vi "ritter sample 1.vi"() -> ()   [LabVIEW 2023]
doc: "Each half second this this program reads the current flow and accumulated volume."
uses:
  Type Definitions/Input Parameters.ctl
  Type Definitions/Full Data.ctl
  Type Definitions/EDU 32 FP Data Cluster.ctl
  <vilib>/Platform/TimedLoop/XDataNode/timing_clust.ctl
  <vilib>/Platform/TimedLoop/XDataNode/nitl_modes.ctl
  <vilib>/Platform/TimedLoop/XDataNode/wakeup.ctl
  <vilib>/platform/TimedLoop/XDataNode/XDataNode.xnode
  <vilib>/Platform/TimedLoop/XDataNode/XDNodeRunTimeDep.lvlib
panel:
  in  "Tab Control 2":enum32{"Page 1", "Page 2"}(tab)
  out "Full Data Set":T1 {"EDU 32 FP- Data"."English"."Gas Flow Rate (cuft/hr)-Raw" format="%.2f"; "EDU 32 FP- Data"."Metric"."Gas Flow Rate (L/hr)-Raw" format="%.2f"}
  in  "Input Parameters":T3={"Barometric Pressure (inHG)"=0.0, "Gas Pressure (in WC)"=0.0, "Gas Temperature (°F)"=0.0, "Standard Pressure (in HG)"=30.0, "Meter Type"=enum."Wet Meter"}
  out "Correction Factor":dbl
  out "Pressure Correction Factor":dbl
  out "Temperature Correction Factor":dbl
  out "Totalized Flow (L)-Corrected":dbl format="%.3f"
  out "Gas Flow Rate (L/hr)-Corrected":dbl format="%.3f"
  in  "Tab Control":enum32{"Main Screen"}(tab)
  in  "Test Point (Nominal)":T4(ring)
  out "Elapsed Time (Hour)":dbl format="%.2f"
  out "Totalization (L) Snapshot 1":dbl format="%.3f"
  out "Gas Flow Rate (L/hr) Snapshot 1":dbl format="%.3f"
  in  "Timer Snapshot 1(Minutes)":dbl=15.0 format="%.2f"
  out "Elapsed Time (Minute)":dbl format="%.2f"
  in  "Ritter VISA":refnum<visa-resource-name>="COM10"
  out "Totalized Flow (L)-Display":dbl format="%.3f"
  out "Gas Flow Rate (L/hr)-Display":dbl format="%.1f"
  out "Gas Flow Rate (L/hr)-Uncorrected-Calibration":dbl format="%.3f"
  in  "Reset":bool
  in  "Exit":bool
  # "STP Correction\nStandard Temperature = 60°F\nStandard Pressure = 30 in HG"
  # "Calculated Correction Factors"
  # "Flow Rate Calibration - Uncorrected"
  # "or"
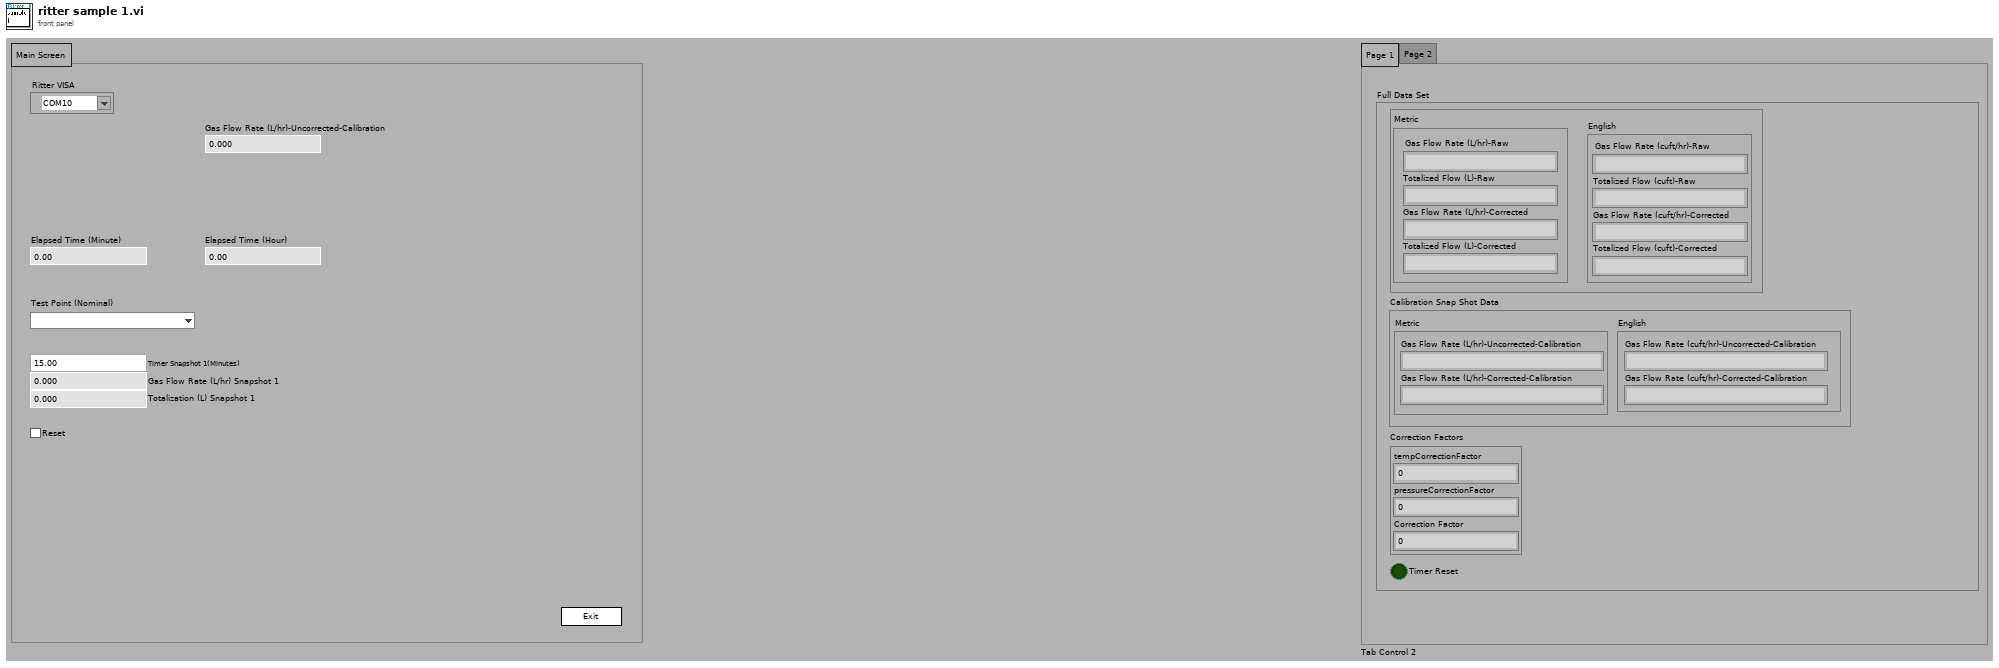
[diagram p1: front panel]
types:
  T1 = typedef "Full Data.ctl" = cluster{"EDU 32 FP- Data":T2, "Calibration Snap Shot Data":cluster{"Metric":cluster{"Gas Flow Rate (L/hr)-Corrected-Calibration":dbl, "Gas Flow Rate (L/hr)-Uncorrected-Calibration":dbl}, "English":cluster{"Gas Flow Rate (cuft/hr)-Corrected-Calibration":dbl, "Gas Flow Rate (cuft/hr)-Uncorrected-Calibration":dbl}}, "Correction Factors":cluster{"tempCorrectionFactor":dbl, "pressureCorrectionFactor":dbl, "Correction Factor":dbl}, "Timer Reset":bool}
  T2 = typedef "EDU 32 FP Data Cluster.ctl" = cluster{"Metric":cluster{"Totalized Flow (L)-Raw":dbl, "Gas Flow Rate (L/hr)-Raw":dbl, "Totalized Flow (L)-Corrected":dbl, "Gas Flow Rate (L/hr)-Corrected":dbl}, "English":cluster{"Totalized Flow (cuft)-Raw":dbl, "Gas Flow Rate (cuft/hr)-Raw":dbl, "Totalized Flow (cuft)-Corrected":dbl, "Gas Flow Rate (cuft/hr)-Corrected":dbl}}
  T3 = typedef "Input Parameters.ctl" = cluster{"Barometric Pressure (inHG)":dbl, "Gas Pressure (in WC)":dbl, "Gas Temperature (°F)":dbl, "Standard Pressure (in HG)":dbl, "Meter Type":enum16{"Wet Meter", "Dry Meter"}}
  T4 = enum16{"", "14 L/hr @ 30 Minutes", "460 L/hr @ 15 Minutes", "900 L/hr @ 15 Minutes", "1100 L/hr @ 15 Minutes", "1100 L/hr @ 100 Minutes", "1300 L/hr @ 15 Minutes"}
  T5 = typedef "XDNodeRunTimeDep.lvlib/timing_clust.ctl" = cluster{"Expected End [f-1]":u64, "Actual End [f-1]":u64, "Finished Late? [f-1]":bool, "Expected End [i-1]":u64, "Actual End [i-1]":u64, "Finished Late? [i-1]":bool, "Expected Start [i]":u64, "Actual Start [i]":u64, "Expected Start [f]":u64, "Actual Start [f]":u64, "Source Name":string, "Structure Name":string, "Period":i64, "Deadline":i64, "Offset":i64, "Start":i64, "Priority":i32, "Timeout":i32, "Mode":T6, "Wakeup Reason":T7, "Error":errorcluster, "Source Type":string, "Secondary Source Type":string, "Global End Time":u64, "Global Start Time":u64, "Frame Duration":u64, "Iteration Duration":u64, "Assigned CPU":i32, "I/O Scan Engine Mode":u32}
  T6 = typedef "XDNodeRunTimeDep.lvlib/nitl_modes.ctl" = enum32{"No Change", "Process missed periods, maintain original phase", "Discard missed periods, maintain original phase", "Process missed periods, ignore original phase", "Discard missed periods, ignore original phase"}
  T7 = typedef "XDNodeRunTimeDep.lvlib/wakeup.ctl" = enum32{"Normal", "Aborted", "Asynchronous wakeup", "Timing source error", "Timed loop error", "Timeout"}
  T8 = enum32{"Invalid", "Standard", "Closed", "Hidden", "Minimized", "Maximized"}
  T9 = enum32{"invalid app kind", "Development System", "Run Time System", "Student Edition", "Embedded LabVIEW", "Evaluation", "Custom"}
  T10 = cluster{"Core":cluster{"Current VI Reference":refnum<vi>, "Close Panel on Exit?":bool}, "Ritter VISA":refnum<visa-resource-name>, "Full Data Set":T1}
  T11 = cluster{"Current VI Reference":refnum<vi>, "Close Panel on Exit?":bool}
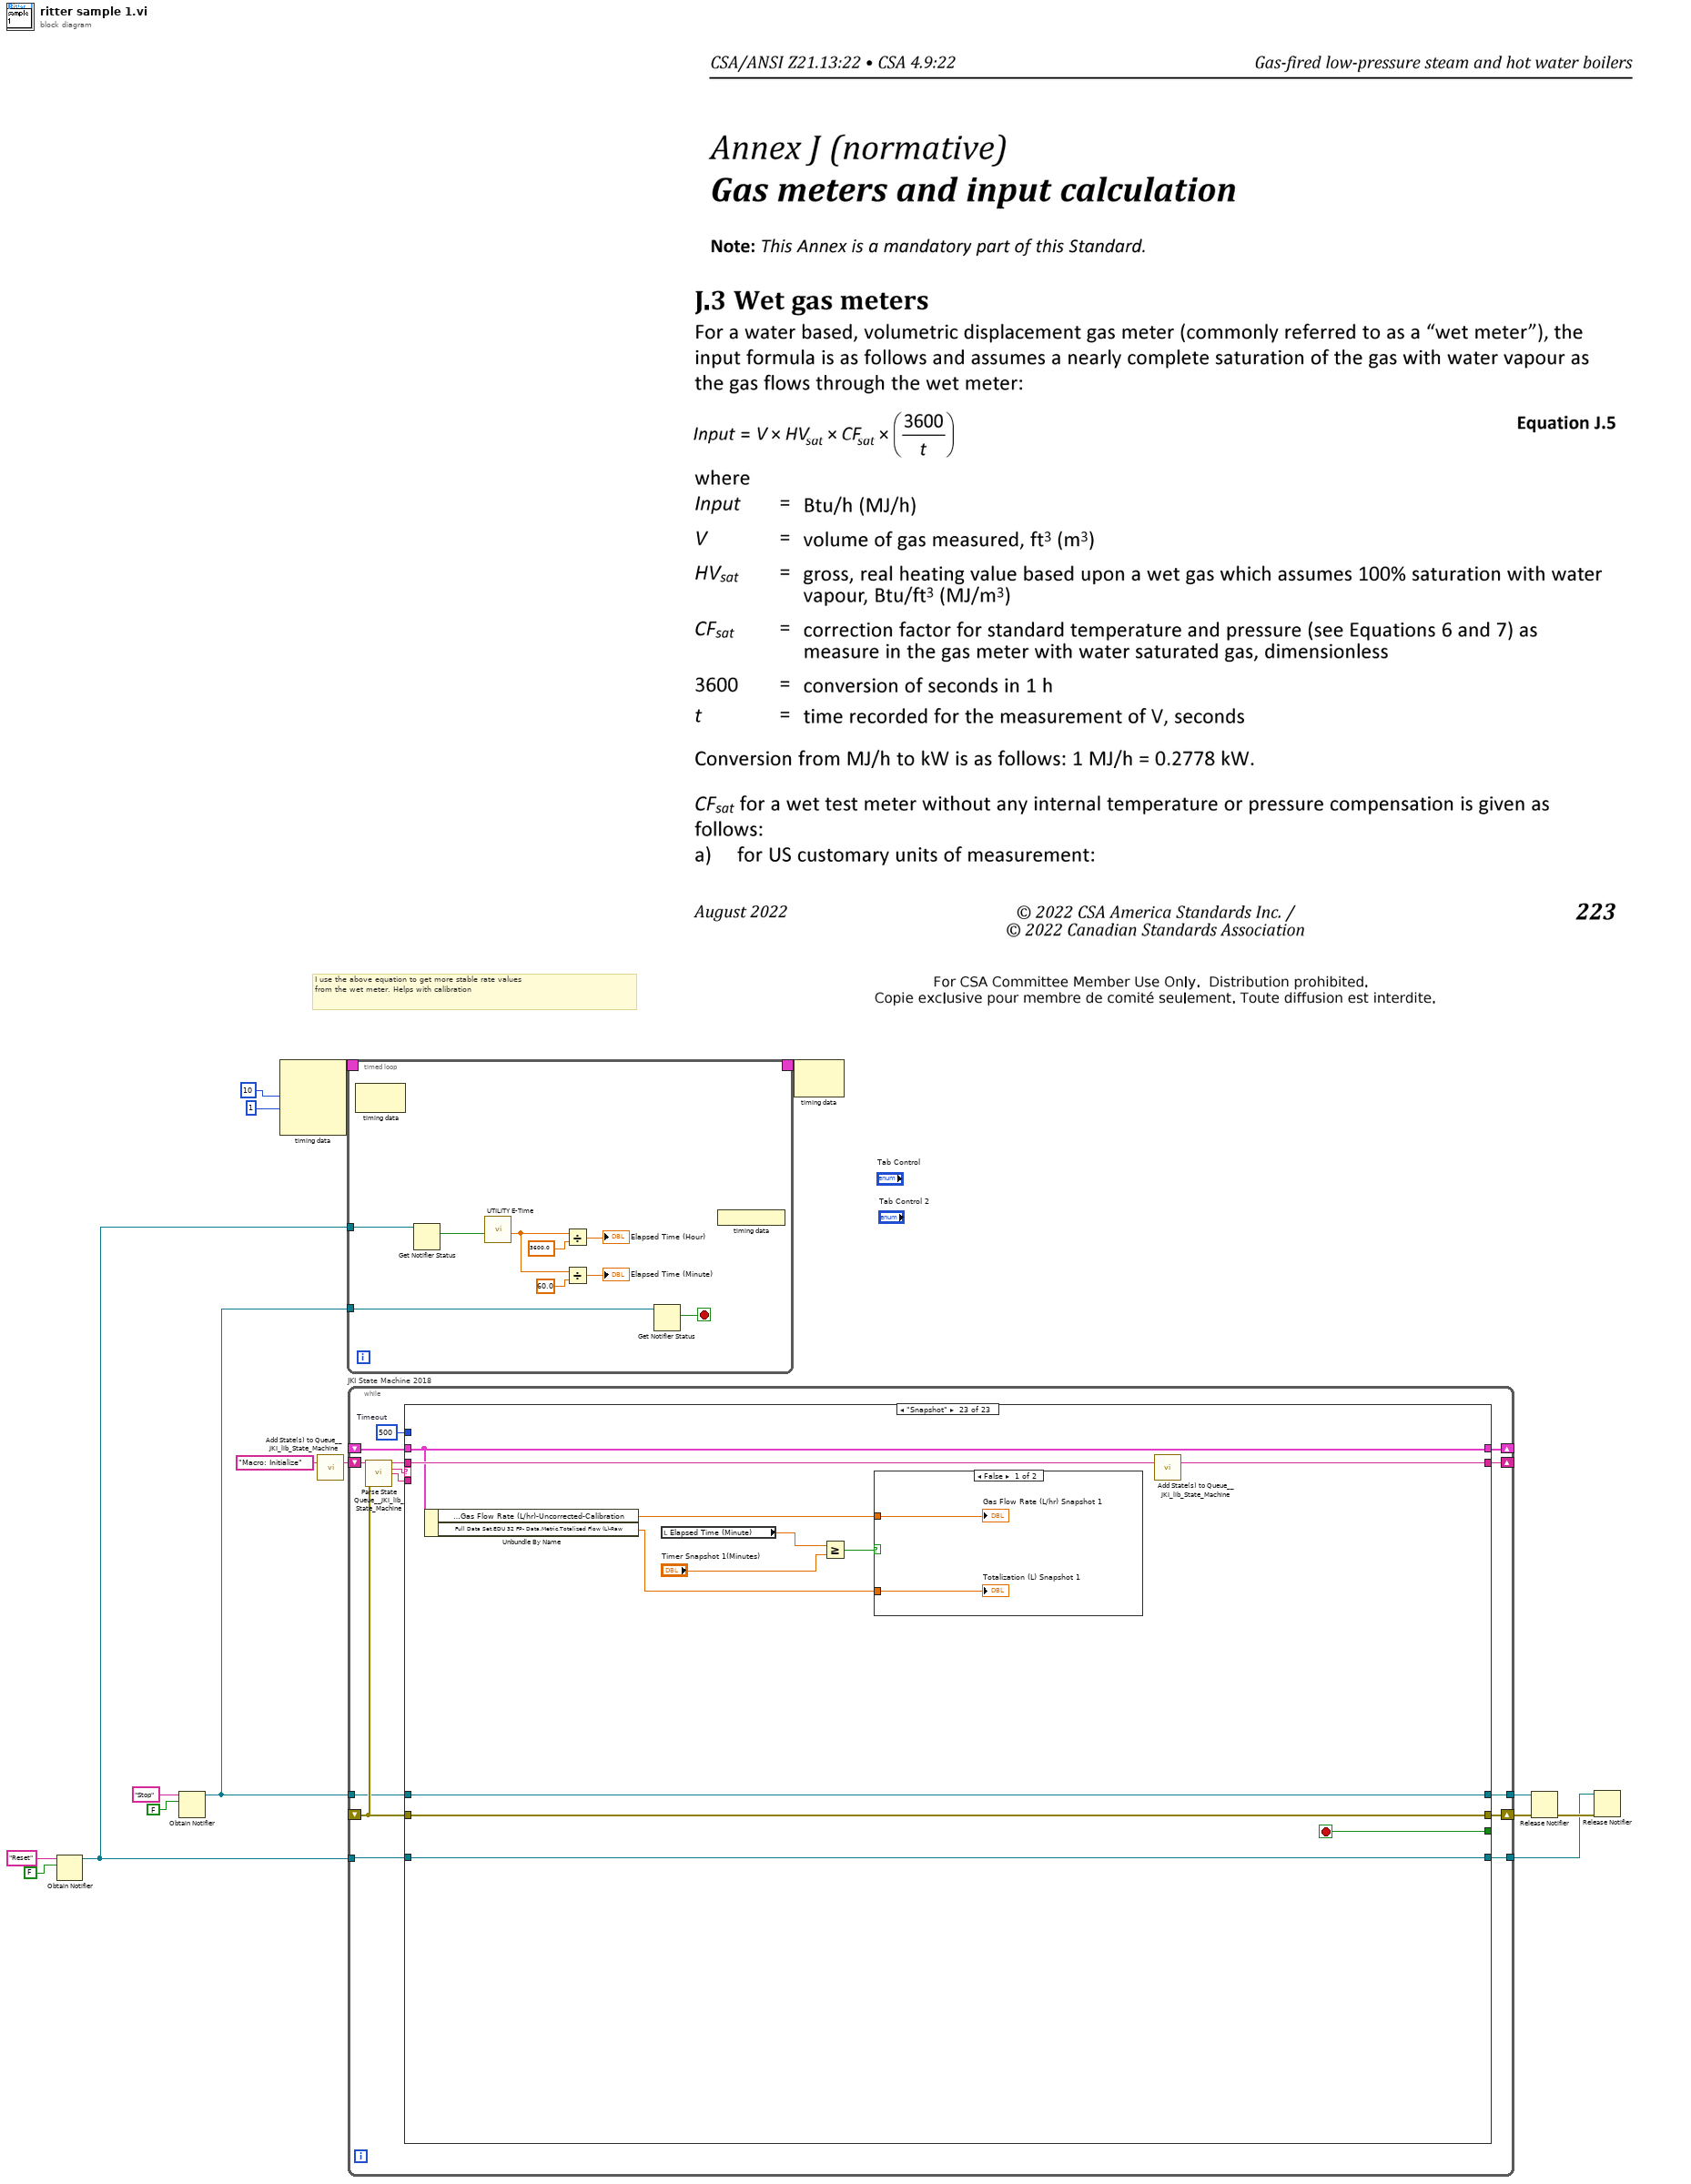
[diagram p0: block diagram]
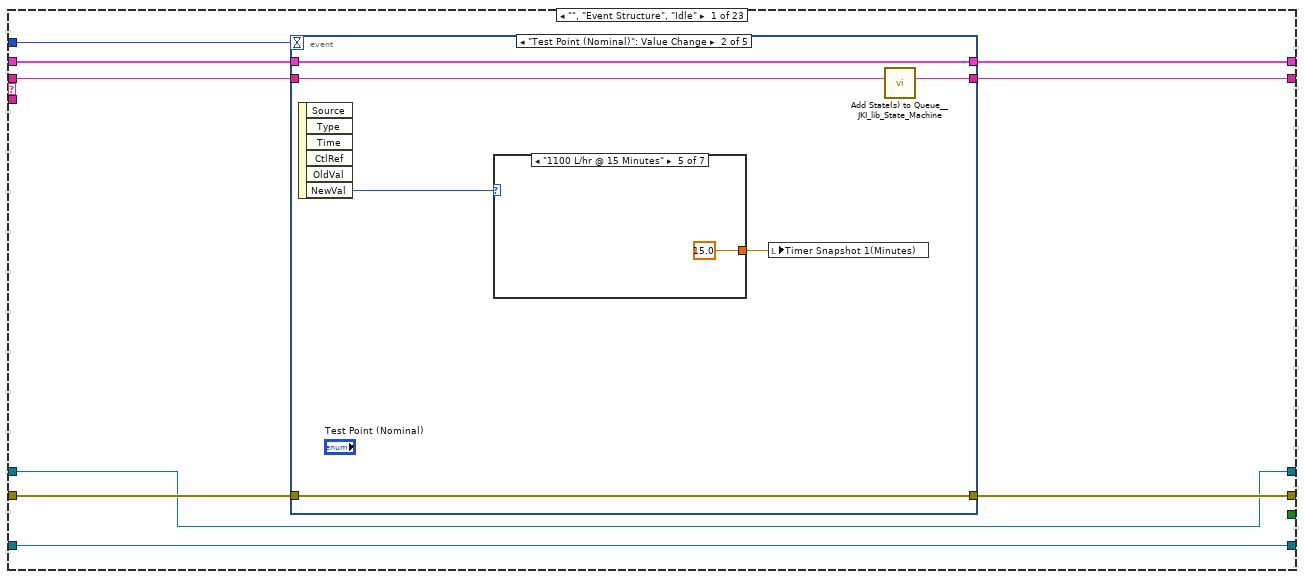
[diagram p2: hidden frame]
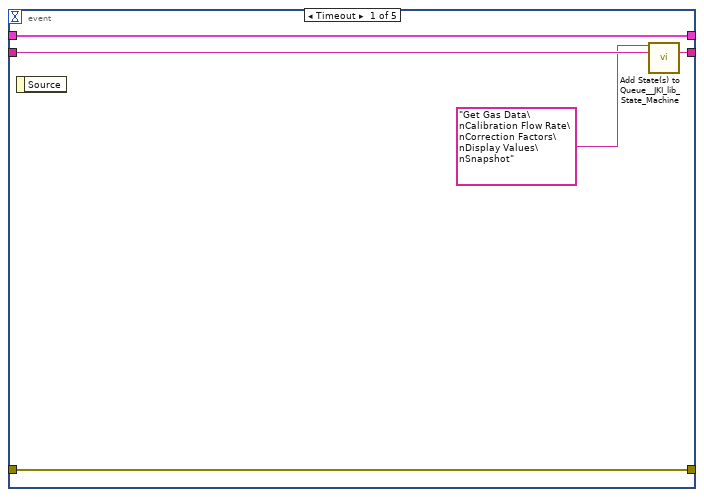
[diagram p3: hidden frame]
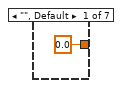
[diagram p4: hidden frame]
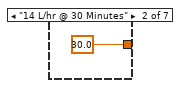
[diagram p5: hidden frame]
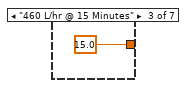
[diagram p6: hidden frame]
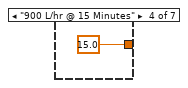
[diagram p7: hidden frame]
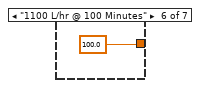
[diagram p8: hidden frame]
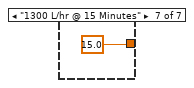
[diagram p9: hidden frame]
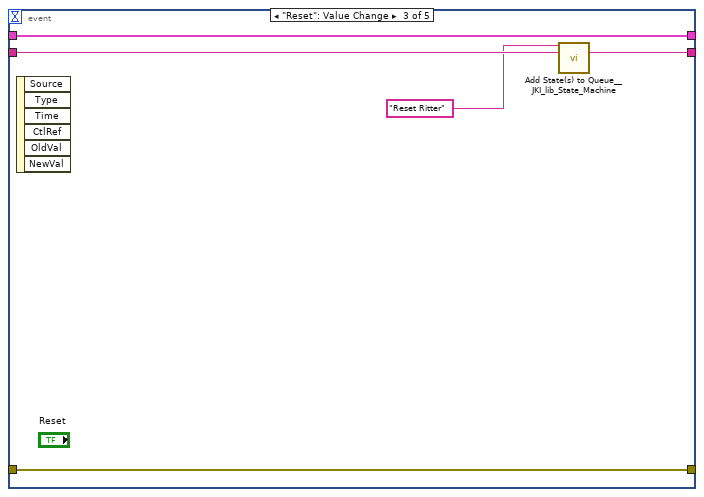
[diagram p10: hidden frame]
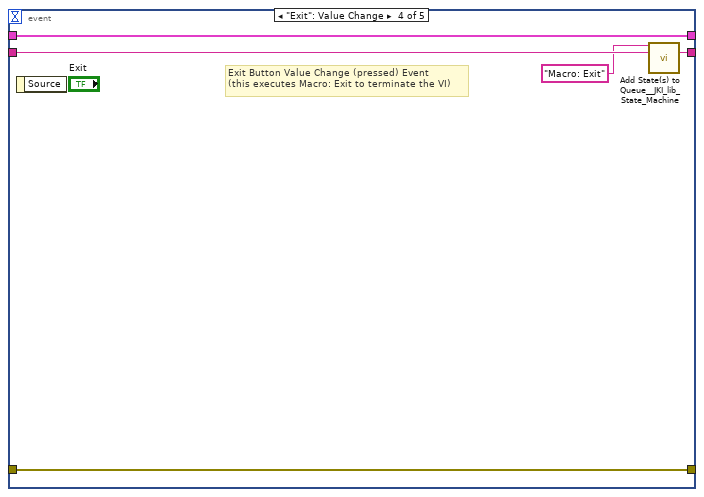
[diagram p11: hidden frame]
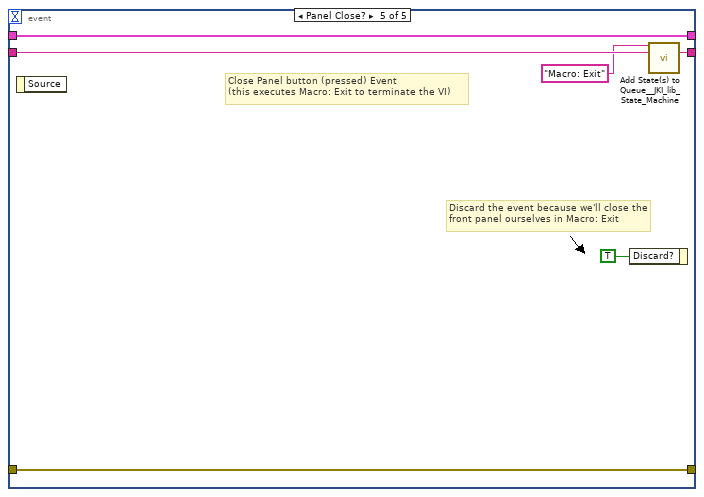
[diagram p12: hidden frame]
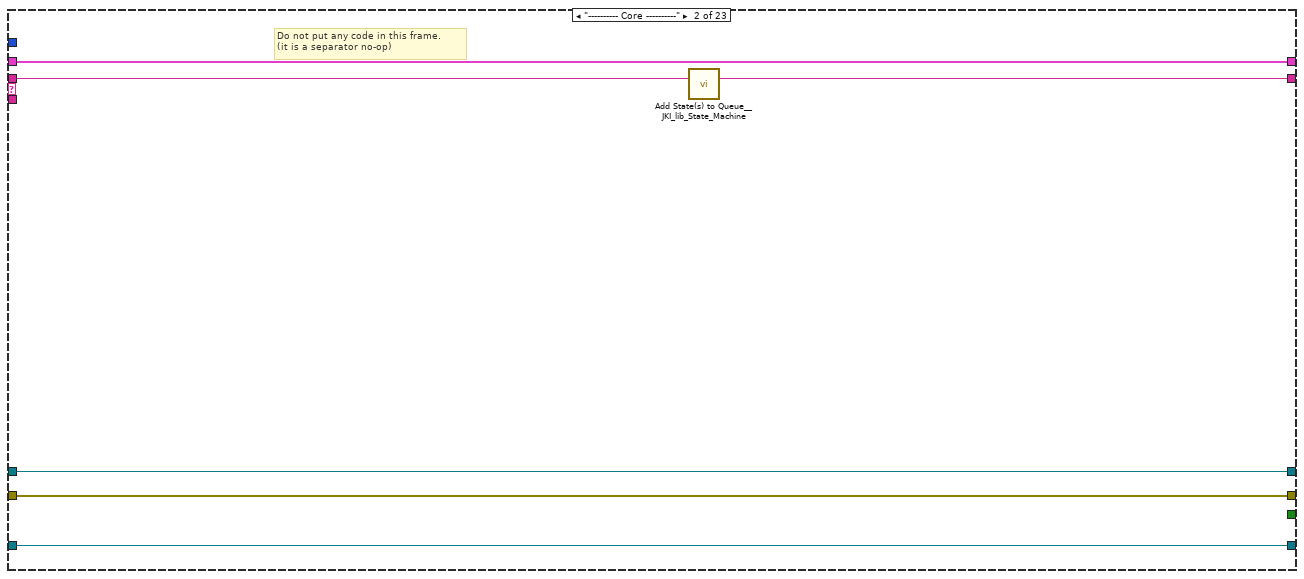
[diagram p13: hidden frame]
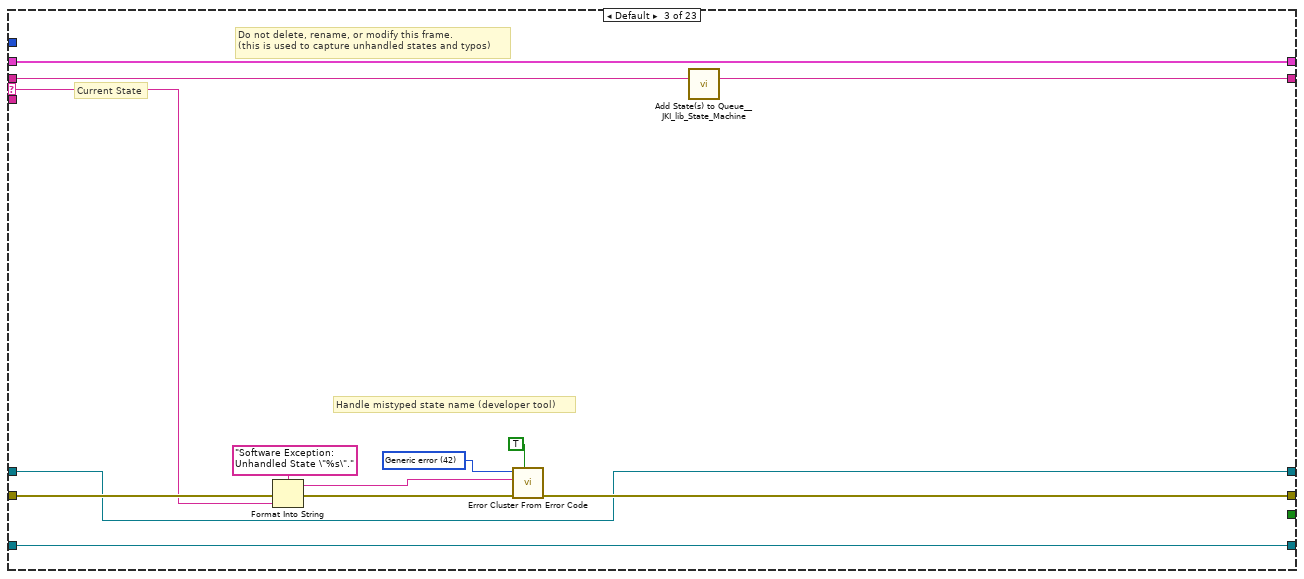
[diagram p14: hidden frame]
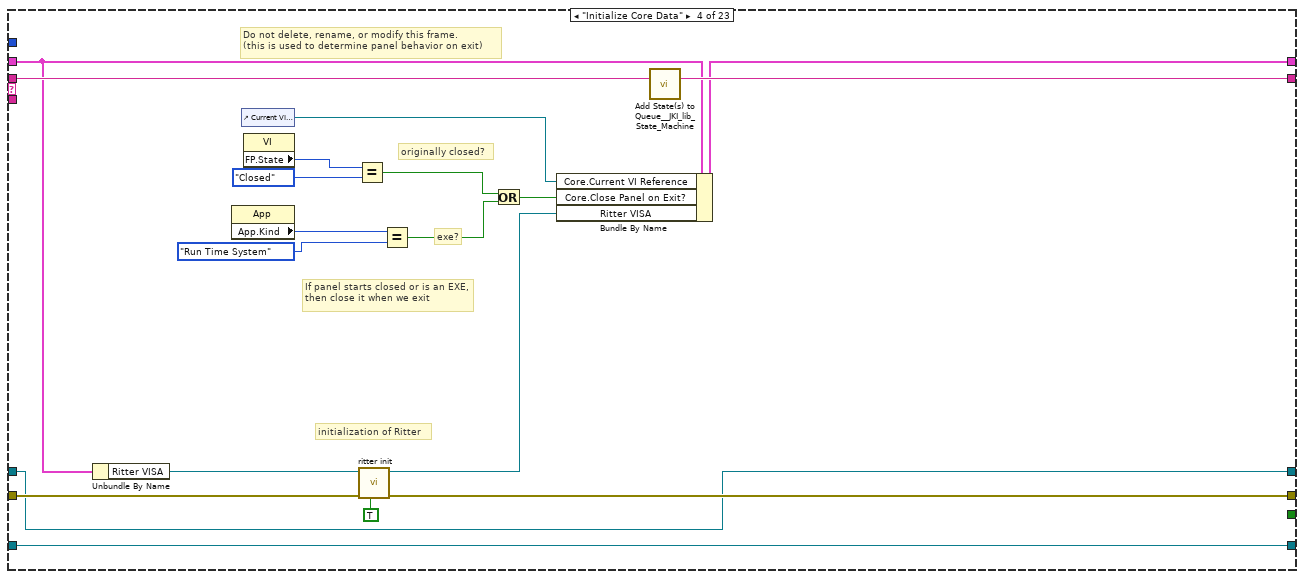
[diagram p15: hidden frame]
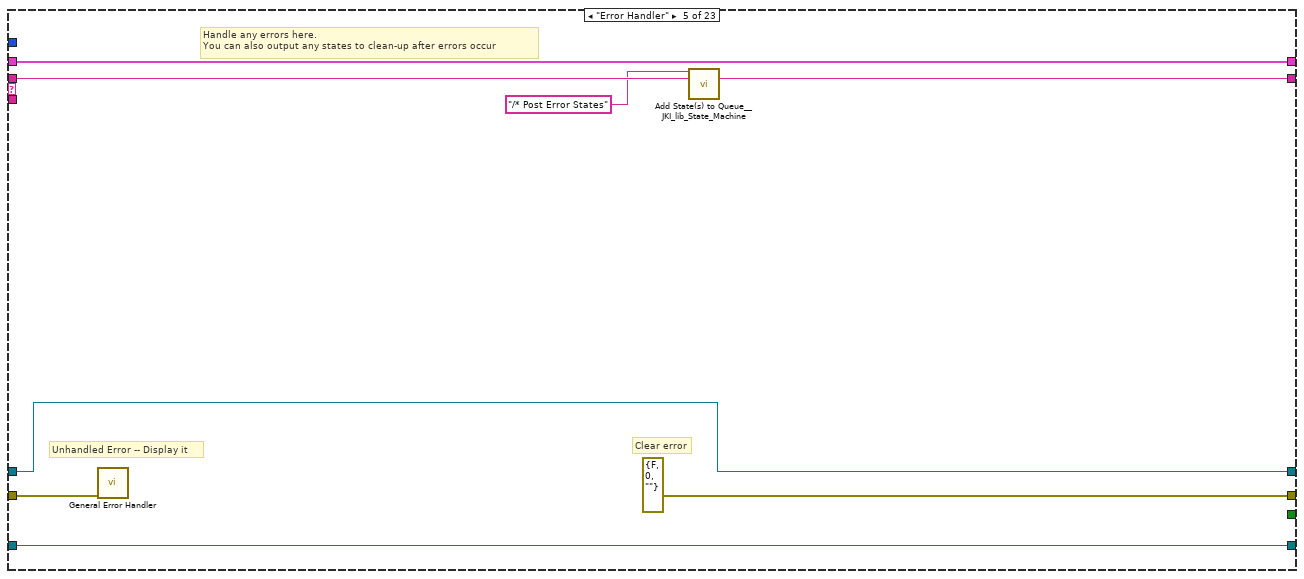
[diagram p16: hidden frame]
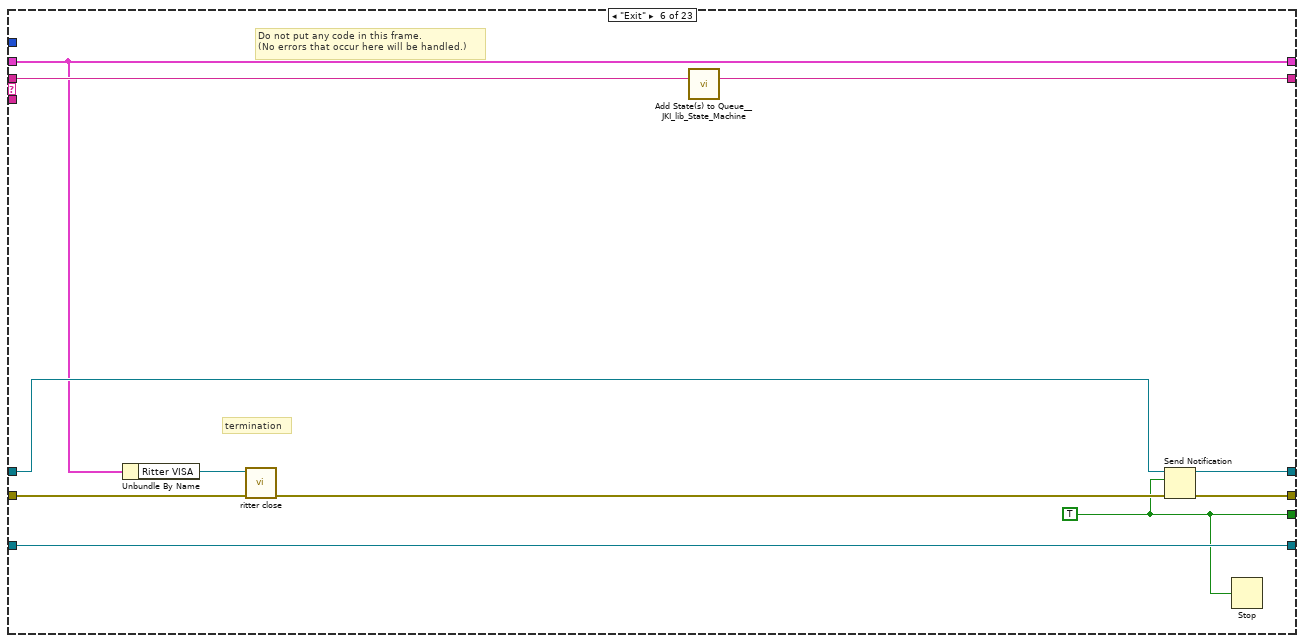
[diagram p17: hidden frame]
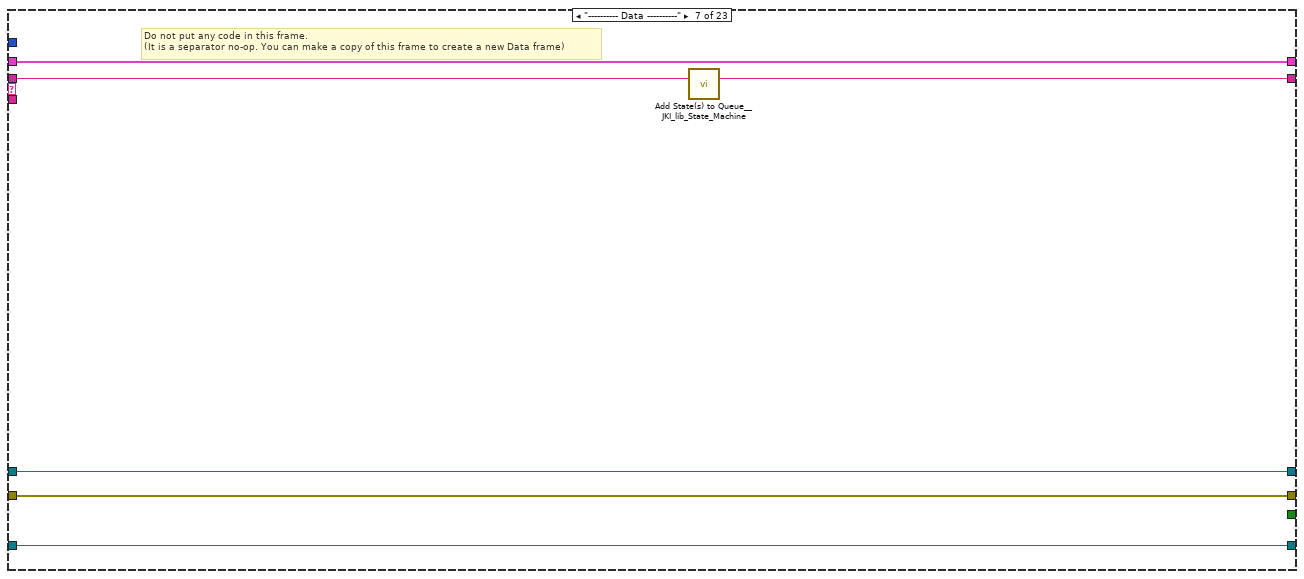
[diagram p18: hidden frame]
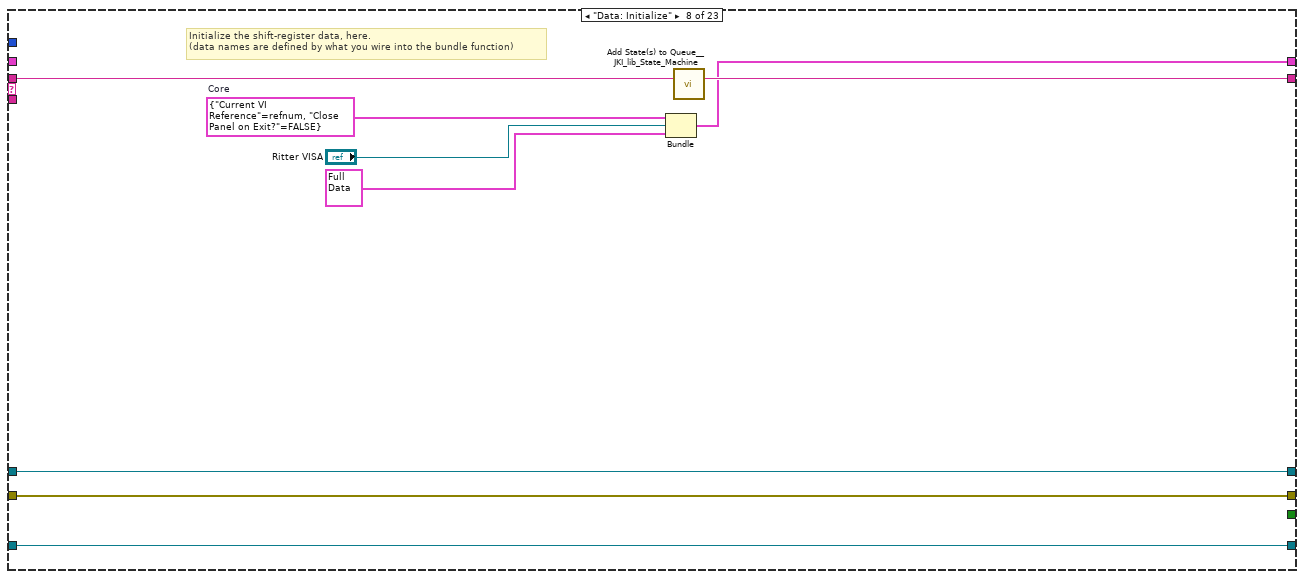
[diagram p19: hidden frame]
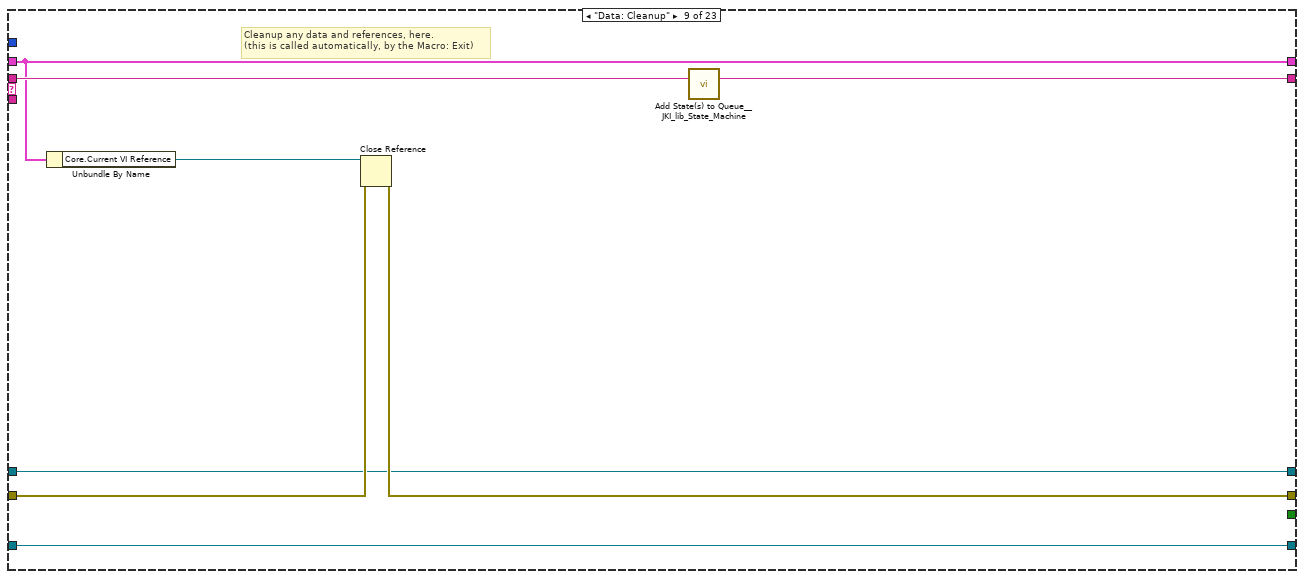
[diagram p20: hidden frame]
diagram:
  # "I use the above equation to get more stable rate values\nfrom the wet meter. Helps with calibration"
  n1 = Obtain Notifier(name (unnamed)="Reset", notification data type=FALSE) -> (notifier out=w3:refnum<notifier>)  [unwired: 2 in, 2 out]
  n2 = Obtain Notifier(name (unnamed)="Stop", notification data type=FALSE) -> (notifier out=w8:refnum<notifier>)  [unwired: 2 in, 2 out]
  n3 = node-c288(u32 10 ("milliseconds to wait"), 1 ("Priority")) -> (w14:T5)  [unwired: 2 in]
  n4 = call <vilib>:"Add State(s) to Queue__JKI_lib_State_Machine.vi"("State(s) in (\"\")"="Macro: Initialize") -> ("States Out"=w10:string)  [unwired: 14 in]
  n5 = timed-loop {
    timing: w14 -> [_]
    timing-out: [_] -> w13
    tunnel: w8 -> [w25]
    tunnel: w3 -> [w18]
    stop <- w22 stop-if-true
    n6 = node-c288() -> ()  [unwired: 1 in, 1 out]
    n7 = Get Notifier Status(notifier=w18) -> (current notification=w17:bool)  [unwired: 1 in, 4 out]
    n8 = call "UTILITY E-Time.vi"("Reset"=w17) -> ("Elapsed Time (sec)"=w19:dbl)  [unwired: 8 in, 2 out]
    n9 = Divide(x=w19, y=3600.0) -> (x/y=→"Elapsed Time (Hour)":dbl)
    n10 = Divide(x=w19, y=60.0) -> (x/y=→"Elapsed Time (Minute)":dbl)
    n11 = Get Notifier Status(notifier=w25) -> (current notification=w22:bool)  [unwired: 1 in, 4 out]
    n12 = node-c288() -> ()  [unwired: 1 out]
  }
  n13 = while "JKI State Machine 2018" {
    shift-right: [w35] -> _
    shift-left: _ -> [w34]
    shift-right: [w38] -> w7
    shift-left: _ -> [w32]
    shift-right: [w37] -> _
    shift-left: w10 -> [w39]
    tunnel: w8 -> [w31]
    tunnel: [w30] -> w6
    tunnel: w3 -> [w29]
    tunnel: [w28] -> w1
    stop <- w36 stop-if-true
    w33 = 500  # Timeout
    n14 = call <vilib>:"Parse State Queue__JKI_lib_State_Machine.vi"("State Queue"=w39, "Error In (no error)"=w32) -> ("Remaining States"=w41:string, "Current State"=w42:string, "Arguments"=w40:string)  [unwired: 11 in]
    n15 = case shown="\"Snapshot\"" w42 {
      selector: w42 -> [_ _ w94 _ _ _ _ _ _ _ _ _ _ _ _ _ _ _ _ _ _ _ _]
      tunnel: w41 -> [w51 w91 w98 w123 w131 w142 w148 w157 w165 w171 w177 w185 w198 w269 w276 w287 w299 w305 w321 w334 w360 w410 w441]
      tunnel: w40 -> [_ _ _ _ _ _ _ _ _ _ _ w180 w192 _ _ _ _ _ _ _ _ _ _]
      tunnel: w34 -> [w49 w88 w96 w109 w128 w136 w145 _ w160 w168 w175 w183 w194 w266 w273 w281 w296 w302 w315 w329 w346 w396 w434]
      tunnel: [w48 w89 w100 w110 errorcluster {"status"=FALSE, "code"=0, "source"=""} ("error out") w140 w146 w154 w161 w169 w174 w181 w195 w267 w274 w283 w297 w303 w313 w330 w356 w407 w438] -> w38
      tunnel: w32 -> [w47 w89 w99 w111 w127 w138 w146 w154 w162 w169 w174 w182 w196 w267 w274 w284 w297 w303 w319 w331 w357 w407 w438]
      tunnel: [w50 w90 w97 w122 w130 w141 w147 w156 w164 w170 w176 w184 w197 w268 w275 w286 w298 w304 w320 w333 w359 w409 w440] -> w37
      tunnel: [_ _ _ _ _ w132 _ _ _ _ _ _ _ _ _ _ _ _ _ _ _ _ _] -> w36
      tunnel: [w46 w88 w96 w121 w128 w136 w145 w155 w160 w168 w175 w183 w194 w266 w273 w280 w296 w302 w314 w328 w345 w395 w434] -> w35
      tunnel: w33 -> [w45 _ _ _ _ _ _ _ _ _ _ _ _ _ _ _ _ _ _ _ _ _ _]
      tunnel: w31 -> [w44 w87 w93 w106 w125 w139 w144 w150 w159 w167 w173 w179 w191 w265 w271 w285 w289 w301 w309 w323 w358 w408 w439]
      tunnel: [w44 w87 w93 w106 w125 w134 w144 w150 w159 w167 w173 w179 w191 w265 w271 w285 w289 w301 w309 w323 w358 w408 w439] -> w30
      tunnel: w29 -> [w43 w86 w92 w105 w124 w133 w143 w149 w158 w166 w172 w178 w190 w264 w270 w278 w288 w300 w306 w322 w335 w394 w437]
      tunnel: [w43 w86 w92 w105 w124 w133 w143 w149 w158 w166 w172 w178 w190 w264 w270 w278 w288 w300 w306 w322 w335 w393 w437] -> w28
      frame "", "Event Structure", "Idle" {
        n16 = event shown="[1] \"Test Point (Nominal)\": Value Change" {
          selector: _ -> [_ _ _ _ _]
          dyn-events: _ -> [_ _ _ _ _]
          timeout: w45 -> [_ _ _ _ _]
          tunnel: w51 -> [w56 w60 w72 w79 w85]
          tunnel: [w55 w61 w71 w78 w84] -> w50
          tunnel: w49 -> [w53 w59 w74 w76 w82]
          tunnel: [w54 w57 w73 w77 w83] -> w48
          tunnel: w47 -> [w54 w57 w73 w77 w83]
          tunnel: [w53 w59 w74 w76 w82] -> w46
          event Timeout {
            n17 = event-data() -> ()  [unwired: 1 in, 1 out]
            n18 = call <vilib>:"Add State(s) to Queue__JKI_lib_State_Machine.vi"("State(s) in Front (\"\")"="Get Gas Data\nCalibration Flow Rate\nCorrection Factors\nDisplay Values\nSnapshot" ("State(s) in Front (\"\")"), "State(s) in (\"\")"=w56) -> ("States Out"=w55:string)  [unwired: 13 in]
          }
          event "Test Point (Nominal)": Value Change {
            n19 = event-data() -> ("NewVal"=w62:T4)  [unwired: 1 in, 5 out]
            n20 = case shown="\"1100 L/hr @ 15 Minutes\"" w62 {
              tunnel: [0.0 30.0 15.0 15.0 15.0 100.0 15.0] -> w58
              frame "", Default {
              }
              frame "14 L/hr @ 30 Minutes" {
              }
              frame "460 L/hr @ 15 Minutes" {
              }
              frame "900 L/hr @ 15 Minutes" {
              }
              frame "1100 L/hr @ 15 Minutes" {
              }
              frame "1100 L/hr @ 100 Minutes" {
              }
              frame "1300 L/hr @ 15 Minutes" {
              }
            }
            n21 = local write "Timer Snapshot 1(Minutes)"(w58) -> ()
            n22 = call <vilib>:"Add State(s) to Queue__JKI_lib_State_Machine.vi"("State(s) in (\"\")"=w60) -> ("States Out"=w61:string)  [unwired: 14 in]
          }
          event "Reset": Value Change {
            n23 = event-data() -> ()  [unwired: 1 in, 6 out]
            n24 = call <vilib>:"Add State(s) to Queue__JKI_lib_State_Machine.vi"("State(s) in Front (\"\")"="Reset Ritter" ("State(s) in Front (\"\")"), "State(s) in (\"\")"=w72) -> ("States Out"=w71:string)  [unwired: 13 in]
          }
          event "Exit": Value Change {
            # "Exit Button Value Change (pressed) Event\n(this executes Macro: Exit to terminate the VI)"
            n25 = event-data() -> ()  [unwired: 1 in, 1 out]
            n26 = call <vilib>:"Add State(s) to Queue__JKI_lib_State_Machine.vi"("State(s) in Front (\"\")"="Macro: Exit", "State(s) in (\"\")"=w79) -> ("States Out"=w78:string)  [unwired: 13 in]
          }
          event Panel Close? {
            # "Discard the event because we'll close the front panel ourselves in Macro: Exit"
            # "Close Panel button (pressed) Event\n(this executes Macro: Exit to terminate the VI)"
            n27 = event-data() -> ()  [unwired: 1 in, 1 out]
            n28 = event-data("Discard?"=TRUE) -> ()  [unwired: 1 in, 1 out]
            n29 = call <vilib>:"Add State(s) to Queue__JKI_lib_State_Machine.vi"("State(s) in Front (\"\")"="Macro: Exit", "State(s) in (\"\")"=w85) -> ("States Out"=w84:string)  [unwired: 13 in]
          }
        }
      }
      frame "---------- Core ----------" {
        # "Do not put any code in this frame.\n(it is a separator no-op)"
        n30 = call <vilib>:"Add State(s) to Queue__JKI_lib_State_Machine.vi"("State(s) in (\"\")"=w91) -> ("States Out"=w90:string)  [unwired: 14 in]
      }
      frame Default {
        w103 = 42 items=["No error", "Argument error", "Memory is full", "Out of zone", "End of file", "File already open", "Generic file I/O error", "File not found", "File permission error", "Disk is full", "Duplicate path", "Too many files open", "System feature not enabled", "Resource file not found", "Cannot add resource", "Resource not found", "Image not found", "Image memory error", "Pen does not exist", "Config type invalid", "Config token not found", "Config parse error", "Config memory error", "Bad external code format", "Bad external code offset", "External code not present", "Null window", "Destroy window error", "Null menu", "Print aborted", "Bad print record", "Print driver error", "Windows error during printing", "Memory error during printing", "Print dialog error", "Generic print error", "Invalid device refnum", "Device not found", "Device parameter error", "Device unit error", "Cannot open device", "Device call aborted", "Generic error", "Cancelled by user", "Object ID too low", "Object ID too high", "Object not in heap", "Unknown heap", "Unknown object (invalid DefProc)", "Unknown object (DefProc not in table)", "Message out of range", "Invalid (null) method", "Unknown message", "Manager call not supported", "Bad address", "Network operation in progress", "Network operation timed out", "Connection is busy", "Network attribute not supported", "Network error", "Address in use", "System out of memory", "Connection aborted", "Connection refused", "Not connected", "Already connected", "Connection closed", "Initialization error (interapplication manager)", "Bad occurrence", "Wait on unbound occurrence handler", "Occurrence queue overflow", "Datalog type conflict", "Unused", "Unrecognized type (interapplication manager)", "Memory corrupt", "Failed to make temporary DLL", "Old CIN version", "Drag socket not found", "Failed to load drop-object", "Failed to register OLE object", "Failed to release OLE object", "Format specifier type mismatch", "Unknown format specifier", "Too few format specifiers", "Too many format specifiers", "Scan failed", "Newer CIN version", "Error converting to variant", "Runtime menu error", "Password tampered", "Variant attribute not found", "Incompatible variant data type", "Event data is not available", "Event Store is not present", "Occurrence is not found", "Event Queue is not created", "Event info is not available", "Refnum passed is NULL", "Error retrieving Class GUID", "Error retrieving CoClass GUID", "Error retrieving TypeLib GUID.", "Bad built application magic bytes.", "Specific driver is different from the specific driver associated with the Logical Name.", "There is no session opened to the class driver.", "Max Error", "MAX - Error with config objects", "MAX - Error loading configuration", "MAX - Group not supported"]
        # "Current State"
        # "Do not delete, rename, or modify this frame.\n(this is used to capture unhandled states and typos)"
        # "Handle mistyped state name (developer tool)"
        n31 = Format Into String(format string="Software Exception: Unhandled State \"%s\"." ("message"), error in=w99, w94) -> (resulting string=w102:string, error out=w101:errorcluster)  [unwired: 1 in]
        n32 = call <vilib>:"Error Cluster From Error Code.vi"("show call chain? (False)"=TRUE, "error in (no error)"=w101, "error message (\"\")"=w102, "error code (0)"=w103) -> ("error out"=w100:errorcluster)  [unwired: 5 in]
        n33 = call <vilib>:"Add State(s) to Queue__JKI_lib_State_Machine.vi"("State(s) in (\"\")"=w98) -> ("States Out"=w97:string)  [unwired: 14 in]
      }
      frame "Initialize Core Data" {
        # "initialization of Ritter"
        # "Do not delete, rename, or modify this frame.\n(this is used to determine panel behavior on exit)"
        # "originally closed?"
        # "exe?"
        # "If panel starts closed or is an EXE, then close it when we exit"
        n34 = Unbundle By Name(w109) -> ("Ritter VISA"=w108:refnum<visa-resource-name>)
        n35 = property class="App"() -> ("App.Kind"=w120:T9)  [unwired: 2 in, 2 out]
        n36 = control-ref of="Current VI Reference"() -> (w116:refnum<vi>)
        n37 = property class="VI"() -> ("FP.State"=w115:T8)  [unwired: 2 in, 2 out]
        n38 = Equal?(x=w115, y=T8."Closed" ("Front Panel Window:State")) -> (x = y?=w113:bool)
        n39 = call "ritter init.vi"("Ritter Gas Drum Meter Enable"=TRUE, "error in (no error)"=w111, "VISA in"=w108) -> ("error out"=w110:errorcluster, "VISA out"=w107:refnum<visa-resource-name>)  [unwired: 7 in]
        n40 = Equal?(x=w120, y=T9."Run Time System" ("Application:Kind")) -> (x = y?=w118:bool)
        n41 = Or(x=w113, y=w118) -> (x .or. y?=w117:bool)
        n42 = Bundle By Name(cluster=w109, "Core.Current VI Reference"=w116, "Core.Close Panel on Exit?"=w117, "Ritter VISA"=w107) -> (w121:T10)
        n43 = call <vilib>:"Add State(s) to Queue__JKI_lib_State_Machine.vi"("State(s) in (\"\")"=w123) -> ("States Out"=w122:string)  [unwired: 14 in]
      }
      frame "Error Handler" {
        # "Unhandled Error -- Display it"
        # "Handle any errors here.\nYou can also output any states to clean-up after errors occur"
        # "Clear error"
        n44 = call <vilib>:"General Error Handler.vi"("error in (no error)"=w127) -> ()  [unwired: 10 in, 5 out]
        n45 = call <vilib>:"Add State(s) to Queue__JKI_lib_State_Machine.vi"("State(s) in Front (\"\")"="/* Post Error States", "State(s) in (\"\")"=w131) -> ("States Out"=w130:string)  [unwired: 13 in]
      }
      frame "Exit" {
        w132 = TRUE
        # "termination"
        # "Do not put any code in this frame.\n(No errors that occur here will be handled.)"
        n46 = Unbundle By Name(w136) -> ("Ritter VISA"=w135:refnum<visa-resource-name>)
        n47 = call "ritter close.vi"("error in (no error)"=w138, "VISA in"=w135) -> ("error out"=w137:errorcluster)  [unwired: 9 in]
        n48 = call <vilib>:"Add State(s) to Queue__JKI_lib_State_Machine.vi"("State(s) in (\"\")"=w142) -> ("States Out"=w141:string)  [unwired: 14 in]
        n49 = Send Notification(notification=w132, notifier=w139, error in (no error)=w137) -> (notifier out=w134:refnum<notifier>, error out=w140:errorcluster)
        n50 = Stop(stop? (T)=w132) -> ()
      }
      frame "---------- Data ----------" {
        # "Do not put any code in this frame.\n(It is a separator no-op. You can make a copy of this frame to create a new Data frame)"
        n51 = call <vilib>:"Add State(s) to Queue__JKI_lib_State_Machine.vi"("State(s) in (\"\")"=w148) -> ("States Out"=w147:string)  [unwired: 14 in]
      }
      frame "Data: Initialize" {
        w153 = T11 {"Current VI Reference"=refnum, "Close Panel on Exit?"=FALSE}  # Core
        # "Initialize the shift-register data, here.\n(data names are defined by what you wire into the bundle function)"
        n52 = Bundle("Core"=w153, "Ritter VISA"="Ritter VISA", "Full Data Set"=T1 {"EDU 32 FP- Data"={"Metric"={"Totalized Flow (L)-Raw"=6.255, "Gas Flow Rate (L/hr)-Raw"=18.0, "Totalized Flow (L)-Corrected"=0.0, "Gas Flow Rate (L/hr)-Corrected"=0.0}, "English"={"Totalized Flow (cuft)-Raw"=0.0, "Gas Flow Rate (cuft/hr)-Raw"=0.0, "Totalized Flow (cuft)-Corrected"=0.0, "Gas Flow Rate (cuft/hr)-Corrected"=0.0}}, "Calibration Snap Shot Data"={"Metric"={"Gas Flow Rate (L/hr)-Corrected-Calibration"=0.0, "Gas Flow Rate (L/hr)-Uncorrected-Calibration"=0.0}, "English"={"Gas Flow Rate (cuft/hr)-Corrected-Calibration"=0.0, "Gas Flow Rate (cuft/hr)-Uncorrected-Calibration"=0.0}}, "Correction Factors"={"tempCorrectionFactor"=0.0, "pressureCorrectionFactor"=0.0, "Correction Factor"=0.0}, "Timer Reset"=FALSE}) -> (w155:T10)  [unwired: 1 in]
        n53 = call <vilib>:"Add State(s) to Queue__JKI_lib_State_Machine.vi"("State(s) in (\"\")"=w157) -> ("States Out"=w156:string)  [unwired: 14 in]
      }
      frame "Data: Cleanup" {
        # "Cleanup any data and references, here.\n(this is called automatically, by the Macro: Exit)"
        n54 = Unbundle By Name(w160) -> ("Core.Current VI Reference"=w163:refnum<vi>)
        n55 = Close Reference(reference=w163, error in (no error)=w162) -> (error out=w161:errorcluster)
        n56 = call <vilib>:"Add State(s) to Queue__JKI_lib_State_Machine.vi"("State(s) in (\"\")"=w165) -> ("States Out"=w164:string)  [unwired: 14 in]
      }
      frame "---------- UI ----------" {
        # "Do not put any code in this frame.\n(It is a separator no-op. You can make a copy of this frame to create a new UI frame)"
        n57 = call <vilib>:"Add State(s) to Queue__JKI_lib_State_Machine.vi"("State(s) in (\"\")"=w171) -> ("States Out"=w170:string)  [unwired: 14 in]
      }
      frame "UI: Initialize" {
        # "Initialize the User Interface, here.\n(this is called automatically, by the Macro: Init)"
        n58 = call <vilib>:"Add State(s) to Queue__JKI_lib_State_Machine.vi"("State(s) in (\"\")"=w177) -> ("States Out"=w176:string)  [unwired: 14 in]
      }
      frame "UI: Cursor Set" {
        # "Argument"
        # "Set and Unset Cursor Busy.\n(Usage: \"UI: Cursor Set >> Busy|Idle\")"
        n59 = case shown="\"Idle\", Default" w180 {
          tunnel: w182 -> [w187 w189]
          tunnel: [w186 w188] -> w181
          frame "Idle", Default {
            n60 = call <vilib>:"Unset Busy.vi"("error in (no error)"=w187) -> ("error out"=w186:errorcluster)  [unwired: 10 in]
          }
          frame "Busy" {
            n61 = call <vilib>:"Set Busy.vi"("error in (no error)"=w189) -> ("error out"=w188:errorcluster)  [unwired: 9 in, 1 out]
          }
        }
        n62 = call <vilib>:"Add State(s) to Queue__JKI_lib_State_Machine.vi"("State(s) in (\"\")"=w185) -> ("States Out"=w184:string)  [unwired: 14 in]
      }
      frame "UI: Front Panel State" {
        # "Argument"
        # "Set Front Panel Open or Closed\n(Usage: \"UI: Front Panel State >> Open|Close\")"
        n63 = Unbundle By Name(w194) -> ("Core.Current VI Reference"=w193:refnum<vi>)
        n64 = case shown="\"Minimize\", \"Minimized\"" w192 {
          tunnel: w196 -> [w204 w219 w230 w243 w256]
          tunnel: [w206 w220 w232 w245 w258] -> w195
          tunnel: w193 -> [w205 w217 w231 w244 w257]
          frame "Open", "Standard", Default {
            w199 = T8."Standard" ("State")
            n65 = property class="VI"(reference=w205, error in=w204) -> (reference out=w202:refnum<vi>, error out=w203:errorcluster, "FP.State"=w201:T8)
            n66 = Not Equal?(x=w201, y=w199) -> (x != y?=w200:bool)
            n67 = case shown="True" w200 {
              tunnel: [w210 w212] -> w206
              tunnel: w203 -> [w209 w212]
              tunnel: w202 -> [w208 _]
              tunnel: w199 -> [w207 _]
              frame True {
                n68 = invoke class="VI" method="FP.Open"(reference=w208, error in=w209, "Activate"=TRUE, "State"=w207) -> (error out=w210:errorcluster)  [unwired: 1 in, 4 out]
              }
              frame False {
              }
            }
          }
          frame "Close", "Closed" {
            n69 = property class="VI"(reference=w217, error in=w219) -> (reference out=w216:refnum<vi>, error out=w218:errorcluster, "FP.State"=w214:T8)
            n70 = Not Equal?(x=w214, y=T8."Closed" ("Front Panel Window:State")) -> (x != y?=w213:bool)
            n71 = case shown="True" w213 {
              tunnel: [w221 w224] -> w220
              tunnel: w218 -> [w221 w223]
              tunnel: w216 -> [_ w222]
              frame False {
              }
              frame True {
                n72 = invoke class="VI" method="FP.Close"(reference=w222, error in=w223) -> (error out=w224:errorcluster)  [unwired: 1 in, 2 out]
              }
            }
          }
          frame "Hidden", "Hide" {
            w225 = T8."Hidden" ("State")
            n73 = property class="VI"(reference=w231, error in=w230) -> (reference out=w228:refnum<vi>, error out=w229:errorcluster, "FP.State"=w227:T8)
            n74 = Not Equal?(x=w227, y=w225) -> (x != y?=w226:bool)
            n75 = case shown="True" w226 {
              tunnel: [w236 w237] -> w232
              tunnel: w229 -> [w235 w237]
              tunnel: w228 -> [w234 _]
              tunnel: w225 -> [w233 _]
              frame True {
                n76 = invoke class="VI" method="FP.Open"(reference=w234, error in=w235, "State"=w233) -> (error out=w236:errorcluster)  [unwired: 2 in, 4 out]
              }
              frame False {
              }
            }
          }
          frame "Minimize", "Minimized" {
            w238 = T8."Minimized" ("State")
            n77 = property class="VI"(reference=w244, error in=w243) -> (reference out=w241:refnum<vi>, error out=w242:errorcluster, "FP.State"=w240:T8)
            n78 = Not Equal?(x=w240, y=w238) -> (x != y?=w239:bool)
            n79 = case shown="True" w239 {
              tunnel: [w249 w250] -> w245
              tunnel: w242 -> [w248 w250]
              tunnel: w241 -> [w247 _]
              tunnel: w238 -> [w246 _]
              frame True {
                n80 = invoke class="VI" method="FP.Open"(reference=w247, error in=w248, "State"=w246) -> (error out=w249:errorcluster)  [unwired: 2 in, 4 out]
              }
              frame False {
              }
            }
          }
          frame "Maximize", "Maximized" {
            w251 = T8."Maximized" ("State")
            n81 = property class="VI"(reference=w257, error in=w256) -> (reference out=w254:refnum<vi>, error out=w255:errorcluster, "FP.State"=w253:T8)
            n82 = Not Equal?(x=w253, y=w251) -> (x != y?=w252:bool)
            n83 = case shown="True" w252 {
              tunnel: [w262 w263] -> w258
              tunnel: w255 -> [w261 w263]
              tunnel: w254 -> [w260 _]
              tunnel: w251 -> [w259 _]
              frame True {
                n84 = invoke class="VI" method="FP.Open"(reference=w260, error in=w261, "State"=w259) -> (error out=w262:errorcluster)  [unwired: 2 in, 4 out]
              }
              frame False {
              }
            }
          }
        }
        n85 = call <vilib>:"Add State(s) to Queue__JKI_lib_State_Machine.vi"("State(s) in (\"\")"=w198) -> ("States Out"=w197:string)  [unwired: 14 in]
      }
      frame "---------- Macro ----------" {
        # "Do not put any code in this frame.\n(It is a separator no-op. You can make a copy of this frame to create a new Macro frame)"
        n86 = call <vilib>:"Add State(s) to Queue__JKI_lib_State_Machine.vi"("State(s) in (\"\")"=w269) -> ("States Out"=w268:string)  [unwired: 14 in]
      }
      frame "Macro: Initialize" {
        w272 = "Data: Initialize\nInitialize Core Data\nUI: Initialize\nUI: Front Panel State >> Open"  # Data: Initialize Initialize Core Data UI: Initialize UI: Front Panel State >> Open
        # "Initialization Macro\n(This is called once, when the VI starts)"
        n87 = call <vilib>:"Add State(s) to Queue__JKI_lib_State_Machine.vi"("State(s) in Front (\"\")"=w272, "State(s) in (\"\")"=w276) -> ("States Out"=w275:string)  [unwired: 13 in]
      }
      frame "Reset Ritter" {
        n88 = Unbundle By Name(w281) -> ("Ritter VISA"=w282:refnum<visa-resource-name>)
        n89 = call "ritter reset.vi"("error in (no error)"=w284, "VISA in"=w282) -> ("error out"=w283:errorcluster)  [unwired: 8 in, 1 out]
        n90 = call <vilib>:"Add State(s) to Queue__JKI_lib_State_Machine.vi"("State(s) in (\"\")"=w287) -> ("States Out"=w286:string)  [unwired: 14 in]
        n91 = local write "Gas Flow Rate (L/hr) Snapshot 1"(0.0 ("Gas Flow Rate (L/hr) Snapshot 1")) -> ()
        n92 = Bundle By Name(cluster=w281, "Full Data Set.Timer Reset"=TRUE ("Full Data Set.Timer Reset Counter")) -> (w280:T10)
      }
      frame "Macro: Exit" {
        # "Exit Macro\n(This is called once, when the VI exits)"
        n93 = Unbundle By Name(w296) -> ("Core.Close Panel on Exit?"=w295:bool)
        n94 = Select(t="UI: Front Panel State >> Close", s=w295, f="") -> (s? t:f=w292:string)
        n95 = call <vilib>:"Add State(s) to Queue__JKI_lib_State_Machine.vi"("State(s) in (\"\")"=w292, "State(s) at Back (\"\")"="Data: Cleanup\nExit") -> ("States Out"=w290:string)  [unwired: 13 in]
        n96 = call <vilib>:"Add State(s) to Queue__JKI_lib_State_Machine.vi"("State(s) in Front (\"\")"=w290, "State(s) in (\"\")"=w299) -> ("States Out"=w298:string)  [unwired: 13 in]
      }
      frame "---------- New Category ----------" {
        # "Template Separator\n(You can make a copy of, or modify, this frame)"
        n97 = call <vilib>:"Add State(s) to Queue__JKI_lib_State_Machine.vi"("State(s) in (\"\")"=w305) -> ("States Out"=w304:string)  [unwired: 14 in]
      }
      frame "Get Gas Data" {
        # "continuously read\nthe current flow"
        # "continuously read the current\naccumulated volume"
        n98 = Unbundle By Name(w315) -> ("Ritter VISA"=w316:refnum<visa-resource-name>)
        n99 = call "ritter flow.vi"("error in (no error)"=w319, "VISA in"=w316) -> ("error out"=w318:errorcluster, "flow (ltr/hr)"=w308:dbl, "flow (cuft/hr)"=w312:dbl, "VISA out"=w317:refnum<visa-resource-name>)  [unwired: 6 in]
        n100 = call "ritter volume.vi"("error in (no error)"=w318, "VISA in"=w317) -> ("error out"=w313:errorcluster, "volume (liters)"=w307:dbl, "volume (cuft)"=w311:dbl, "VISA out"=w310:refnum<visa-resource-name>)  [unwired: 6 in]
        n101 = call <vilib>:"Add State(s) to Queue__JKI_lib_State_Machine.vi"("State(s) in (\"\")"=w321) -> ("States Out"=w320:string)  [unwired: 14 in]
        n102 = Bundle By Name(cluster=w315, "Full Data Set.EDU 32 FP- Data.English.Gas Flow Rate (cuft/hr)-Raw"=w312, "Full Data Set.EDU 32 FP- Data.Metric.Gas Flow Rate (L/hr)-Raw"=w308, "Full Data Set.EDU 32 FP- Data.English.Totalized Flow (cuft)-Raw"=w311, "Full Data Set.EDU 32 FP- Data.Metric.Totalized Flow (L)-Raw"=w307, "Ritter VISA"=w310) -> (w314:T10)
      }
      frame "Calibration Flow Rate" {
        # "Using the totalized flow, differentiate it\nto get the rate. This is more stable for calibration.\nParticularly at low flow rates"
        n103 = Unbundle By Name(w329) -> ("Full Data Set.EDU 32 FP- Data.English.Totalized Flow (cuft)-Raw"=w325:dbl, "Full Data Set.EDU 32 FP- Data.Metric.Totalized Flow (L)-Raw"=w324:dbl)
        n104 = local read "Elapsed Time (Hour)"() -> (w332:dbl)
        n105 = call "Ritter Derivative of Totalizer.vi"("error in (no error)"=w331, "volume (liters)"=w324, "volume (cuft)"=w325, "timer (hours)"=w332) -> ("error out"=w330:errorcluster, "Gas Flow Rate (L/hr)-Uncorrected"=w326:dbl, "Gas Flow Rate (cuft/hr)-Uncorrected"=w327:dbl)  [unwired: 5 in]
        n106 = Bundle By Name(cluster=w329, "Full Data Set.Calibration Snap Shot Data.English.Gas Flow Rate (cuft/hr)-Uncorrected-Calibration"=w327, "Full Data Set.Calibration Snap Shot Data.Metric.Gas Flow Rate (L/hr)-Uncorrected-Calibration"=w326) -> (w328:T10)
        n107 = call <vilib>:"Add State(s) to Queue__JKI_lib_State_Machine.vi"("State(s) in (\"\")"=w334) -> ("States Out"=w333:string)  [unwired: 14 in]
      }
      frame "Correction Factors" {
        n108 = Unbundle By Name(w346) -> ("Full Data Set.Calibration Snap Shot Data.English.Gas Flow Rate (cuft/hr)-Uncorrected-Calibration"=w347:dbl, "Full Data Set.EDU 32 FP- Data.English.Gas Flow Rate (cuft/hr)-Raw"=w349:dbl, "Full Data Set.EDU 32 FP- Data.English.Totalized Flow (cuft)-Raw"=w348:dbl)
        n109 = Unbundle By Name("Input Parameters") -> ("Meter Type"=w354:enum16{"Wet Meter", "Dry Meter"}, "Standard Pressure (in HG)"=w353:dbl, "Gas Temperature (°F)"=w352:dbl, "Barometric Pressure (inHG)"=w351:dbl, "Gas Pressure (in WC)"=w350:dbl)
        n110 = case shown="\"Wet Meter\", Default" w354 {
          tunnel: w357 -> [w375 w392]
          tunnel: [w376 w390] -> w356
          tunnel: w353 -> [w373 w385]
          tunnel: w352 -> [w372 w386]
          tunnel: w351 -> [w371 w384]
          tunnel: w350 -> [w370 w383]
          tunnel: w349 -> [w369 w389]
          tunnel: w348 -> [w368 w388]
          tunnel: w347 -> [w367 w387]
          tunnel: [w365 w382] -> w343
          tunnel: [w364 w381] -> w342
          tunnel: [w366 w380] -> w344
          tunnel: [w362 w379] -> w341
          tunnel: [w361 w378] -> w339
          tunnel: [w363 w377] -> w336
          frame "Dry Meter" {
            # "This is the correction for the \ndifferentiated flow rate"
            # "This is the full correction"
            n111 = call "Ritter Dry Meter Calculations.vi"("Heise Barometric Pressure (inHG)"=w371, "Gas Temperature (F)"=w372, "standardPressure (in HG)"=w373, "Gas Pressure (in WC)"=w370, "Gas Flow Rate (cuft/hr)-Uncorrected"=w369, "Totalized Flow (cuft)-Uncorrected"=w368, "error in (no error)"=w375) -> ("CFdry"=w366:dbl, "tempCorrectionFactor"=w365:dbl, "pressureCorrectionFactor"=w364:dbl, "gasFlowRate"=w362:dbl, "gasVolume"=w361:dbl, "error out"=w374:errorcluster)  [unwired: 1 in, 2 out]
            n112 = call "Ritter Dry Meter Calculations.vi"("Heise Barometric Pressure (inHG)"=w371, "Gas Temperature (F)"=w372, "standardPressure (in HG)"=w373, "Gas Pressure (in WC)"=w370, "Gas Flow Rate (cuft/hr)-Uncorrected"=w367, "error in (no error)"=w374) -> ("gasFlowRate"=w363:dbl, "error out"=w376:errorcluster)  [unwired: 2 in, 6 out]
          }
          frame "Wet Meter", Default {
            # "This is the correction for the \ndifferentiated flow rate"
            # "This is the full correction"
            n113 = call "Ritter Wet Meter Calculations.vi"("Heise Barometric Pressure (inHG)"=w384, "Gas Pressure (in WC)"=w383, "Gas Flow Rate (cuft/hr)-Uncorrected"=w389, "Totalized Flow (cuft)-Uncorrected"=w388, "error in (no error)"=w392, "Gas Temperature (F)"=w386, "standardPressure (in HG)"=w385) -> ("CFsat"=w380:dbl, "tempCorrectionFactor"=w382:dbl, "pressureCorrectionFactor"=w381:dbl, "gasFlowRate"=w379:dbl, "gasVolume"=w378:dbl, "error out"=w391:errorcluster)  [unwired: 4 in, 3 out]
            n114 = call "Ritter Wet Meter Calculations.vi"("Heise Barometric Pressure (inHG)"=w384, "Gas Pressure (in WC)"=w383, "Gas Flow Rate (cuft/hr)-Uncorrected"=w387, "error in (no error)"=w391, "Gas Temperature (F)"=w386, "standardPressure (in HG)"=w385) -> ("gasFlowRate"=w377:dbl, "error out"=w390:errorcluster)  [unwired: 5 in, 7 out]
          }
        }
        n115 = call <vilib>:"Add State(s) to Queue__JKI_lib_State_Machine.vi"("State(s) in (\"\")"=w360) -> ("States Out"=w359:string)  [unwired: 14 in]
        n116 = expression code="x/0.0353147"(w336) -> (w337:dbl)
        n117 = expression code="x/0.0353147"(w341) -> (w340:dbl)
        n118 = expression code="x/0.0353147"(w339) -> (w338:dbl)
        n119 = Bundle By Name(cluster=w346, "Full Data Set.Calibration Snap Shot Data.Metric.Gas Flow Rate (L/hr)-Corrected-Calibration"=w337, "Full Data Set.Calibration Snap Shot Data.English.Gas Flow Rate (cuft/hr)-Corrected-Calibration"=w336, "Full Data Set.Correction Factors.Correction Factor"=w344, "Full Data Set.Correction Factors.tempCorrectionFactor"=w343, "Full Data Set.Correction Factors.pressureCorrectionFactor"=w342, "Full Data Set.EDU 32 FP- Data.English.Gas Flow Rate (cuft/hr)-Corrected"=w341, "Full Data Set.EDU 32 FP- Data.English.Totalized Flow (cuft)-Corrected"=w339, "Full Data Set.EDU 32 FP- Data.Metric.Gas Flow Rate (L/hr)-Corrected"=w340, "Full Data Set.EDU 32 FP- Data.Metric.Totalized Flow (L)-Corrected"=w338) -> (w345:T10)
      }
      frame "Display Values" {
        n120 = Unbundle By Name(w396) -> ("Full Data Set.Correction Factors.tempCorrectionFactor"=→"Temperature Correction Factor":dbl, "Full Data Set.Correction Factors.pressureCorrectionFactor"=→"Correction Factor":dbl, "Full Data Set.Correction Factors.Correction Factor"=→"Pressure Correction Factor":dbl, "Full Data Set.EDU 32 FP- Data.Metric.Gas Flow Rate (L/hr)-Corrected"=→"Gas Flow Rate (L/hr)-Corrected":dbl, "Full Data Set.EDU 32 FP- Data.Metric.Totalized Flow (L)-Corrected"=→"Totalized Flow (L)-Corrected":dbl, "Full Data Set.Calibration Snap Shot Data.Metric.Gas Flow Rate (L/hr)-Uncorrected-Calibration"=→"Gas Flow Rate (L/hr)-Uncorrected-Calibration":dbl, "Full Data Set.EDU 32 FP- Data.Metric.Gas Flow Rate (L/hr)-Raw"=→"Gas Flow Rate (L/hr)-Display":dbl, "Full Data Set.EDU 32 FP- Data.Metric.Totalized Flow (L)-Raw"=→"Totalized Flow (L)-Display":dbl, "Full Data Set"=w397:T1, "Full Data Set.Timer Reset"=w398:bool)
        "Full Data Set" <- w397
        n121 = case shown="False" w398 {
          tunnel: w397 -> [_ w422]
          tunnel: w396 -> [w414 w418]
          tunnel: [w414 w417] -> w395
          tunnel: w394 -> [w412 w416]
          tunnel: [w411 w415] -> w393
          frame False {
            n122 = Send Notification(notification=FALSE, notifier=w412) -> (notifier out=w411:refnum<notifier>)  [unwired: 1 in, 1 out]
          }
          frame True {
            n123 = Unbundle By Name(w422) -> ("EDU 32 FP- Data.Metric.Totalized Flow (L)-Raw"=w421:dbl)
            n124 = Greater?(x=w421, y=0.001) -> (0:w419:bool)
            n125 = case shown="True" w419 {
              tunnel: w418 -> [w424 w430]
              tunnel: [w424 w429] -> w417
              tunnel: w416 -> [w423 w427]
              tunnel: [w423 w425] -> w415
              frame False {
              }
              frame True {
                n126 = Bundle By Name(cluster=w430, "Full Data Set.Timer Reset"=FALSE ("Full Data Set.Timer Reset Counter")) -> (w429:T10)
                n127 = Send Notification(notification=TRUE, notifier=w427) -> (notifier out=w425:refnum<notifier>)  [unwired: 1 in, 1 out]
              }
            }
          }
        }
        n128 = call <vilib>:"Add State(s) to Queue__JKI_lib_State_Machine.vi"("State(s) in (\"\")"=w410) -> ("States Out"=w409:string)  [unwired: 14 in]
      }
      frame "Snapshot" {
        n129 = Unbundle By Name(w434) -> ("Full Data Set.Calibration Snap Shot Data.Metric.Gas Flow Rate (L/hr)-Uncorrected-Calibration"=w432:dbl, "Full Data Set.EDU 32 FP- Data.Metric.Totalized Flow (L)-Raw"=w431:dbl)
        n130 = local read "Elapsed Time (Minute)"() -> (w433:dbl)
        n131 = Greater Or Equal?(x=w433, y="Timer Snapshot 1(Minutes)") -> (x >= y?=w435:bool)
        n132 = case shown="False" w435 {
          tunnel: w432 -> [w443 _]
          tunnel: w431 -> [w442 _]
          frame False {
            "Gas Flow Rate (L/hr) Snapshot 1" <- w443
            "Totalization (L) Snapshot 1" <- w442
          }
          frame True {
          }
        }
        n133 = call <vilib>:"Add State(s) to Queue__JKI_lib_State_Machine.vi"("State(s) in (\"\")"=w441) -> ("States Out"=w440:string)  [unwired: 14 in]
      }
    }
  }
  n134 = node-c288(w13) -> ()  [unwired: 1 out]
  n135 = Release Notifier(notifier=w6, error in (no error)=w7) -> (error out=w2:errorcluster)  [unwired: 1 in, 2 out]
  n136 = Release Notifier(notifier=w1, error in (no error)=w2) -> ()  [unwired: 1 in, 3 out]
